vi "Lock Control in The Center.vi"(6 "offset":cluster{"x":i32, "y":i32}, 8 "error in (no error)":errorcluster, 11 "TabControl in":refnum<vi>) -> (0 "error out":errorcluster)   [LabVIEW 2017]
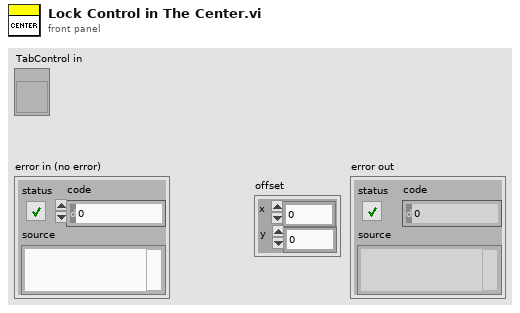
[diagram p1: front panel]
types:
  T1 = typedef "LVBoundsTypeDef.ctl" = cluster{"Width":u32, "Height":u32}
  T2 = typedef "LVPositionTypeDef.ctl" = cluster{"Left":i32, "Top":i32}
  T3 = cluster{"left":i16, "top":i16, "right":i16, "bottom":i16}
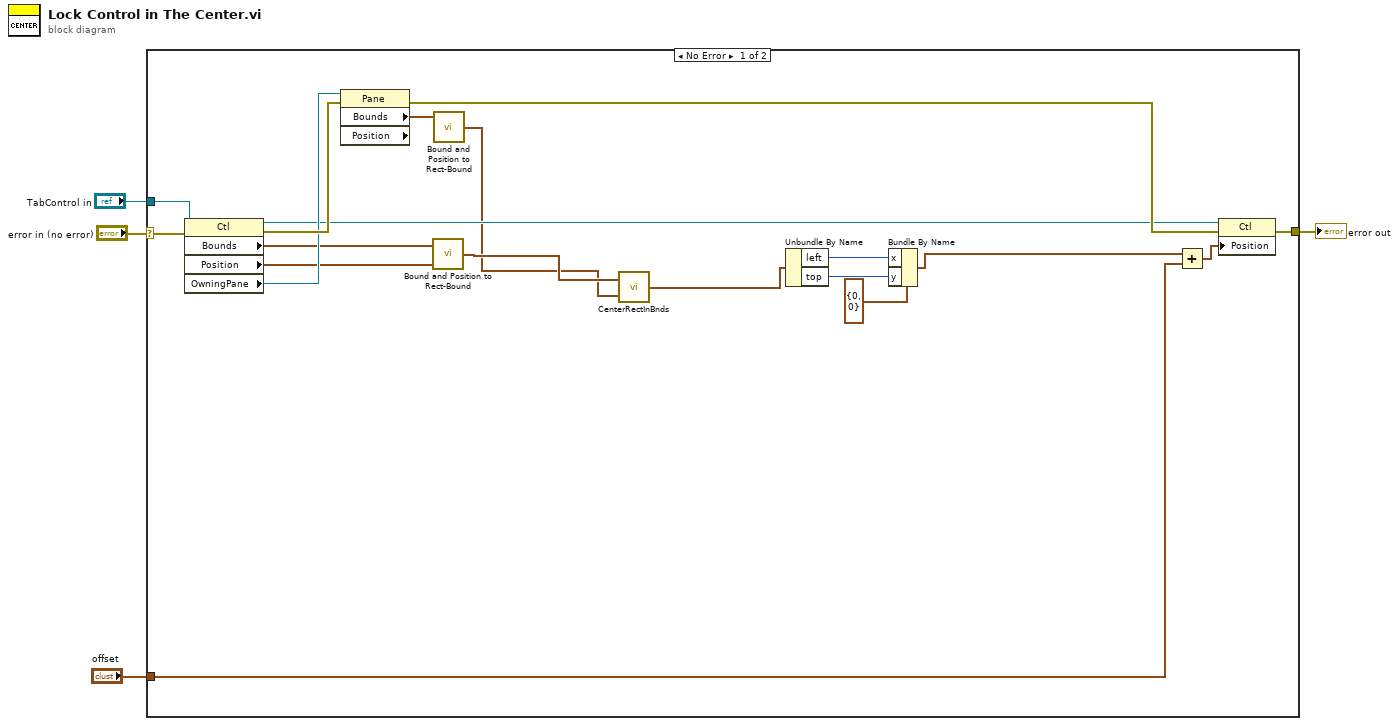
[diagram p0: block diagram]
diagram:
  n1 = case shown="No Error" "error in (no error)" {
    selector: "error in (no error)" -> [w12 w24]
    tunnel: "TabControl in" -> [w14 _]
    tunnel: [w13 w24] -> w3
    tunnel: "offset" -> [w9 _]
    frame No Error {
      n2 = property on="Property Node" class="Ctl"(reference=w14, error in=w12) -> (reference out=w20:refnum<vi>, error out=w22:errorcluster, "Bounds"=w15:T1, "Position"=w16:T2, "OwningPane"=w21:refnum<vi>)
      n3 = property on="Property Node" class="Pane" props=["Bounds", "Position"](reference=w21, error in=w22) -> (error out=w23:errorcluster, "Bounds"=w17:T1)  [unwired: 2 out]
      n4 = call "Bound and Position to Rect-Bound.vi"("Position"=w16, "Bounds"=w15) -> ("Rect Bound"=w19:T3)  [unwired: 3 in]
      n5 = call "Bound and Position to Rect-Bound.vi"("Bounds"=w17) -> ("Rect Bound"=w18:T3)  [unwired: 4 in]
      n6 = call <vilib>:"CenterRectInBnds.vi"("bounds"=w18, "rect"=w19) -> ("centered rect"=w8:T3)
      n7 = Unbundle By Name(w8) -> ("left"=w6:i16, "top"=w7:i16)
      n8 = Bundle By Name(cluster=cluster{"x":i32, "y":i32} {"x"=0, "y"=0} ("Point"), "x"=w6, "y"=w7) -> (w11:cluster{"x":i32, "y":i32})
      n9 = Add(x=w11, y=w9) -> (x+y=w10:cluster{"x":i32, "y":i32})
      n10 = property on="Property Node" class="Ctl"(reference=w20, error in=w23, "Position"=w10) -> (error out=w13:errorcluster)  [unwired: 1 out]
    }
    frame Error {
    }
  }
  "error out" <- w3
